vi "Observer.vi"(8 "Tau":dbl[](array[numeric]), 9 "y":dbl[](array[numeric]), 11 "OBS_K":dbl[](array[numeric])) -> (2 "q_hat":T1)   [LabVIEW 2019]
uses:
  <vilib>/Analysis/Matrix/Datatypes/RealMatrix.ctl
  <vilib>/Analysis/Matrix/NI_Matrix.lvlib
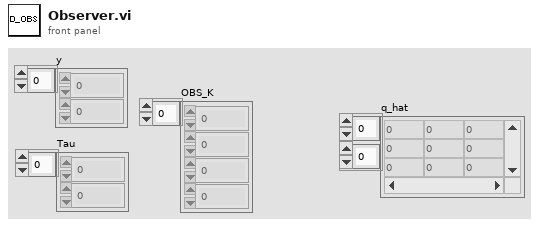
[diagram p1: front panel]
types:
  T1 = typedef "NI_Matrix.lvlib/RealMatrix.ctl" = dbl[][]
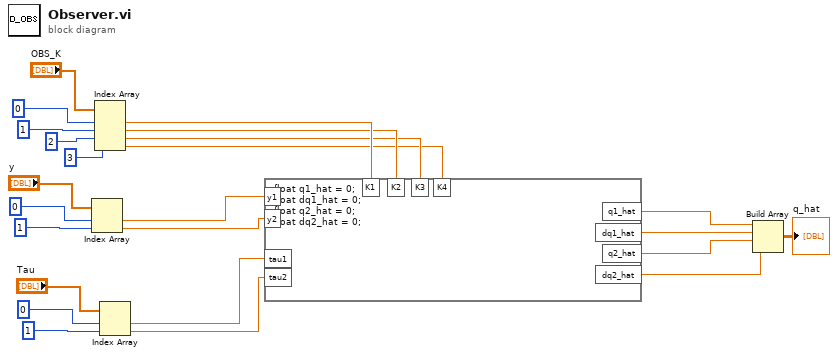
[diagram p0: block diagram]
diagram:
  n1 = Index Array(array="y", index #1=0 ("index (row)"), index #2=1 ("index (col)")) -> (element #1=w2:dbl, element #2=w1:dbl)
  n2 = Index Array(array="OBS_K", index #1=0 ("index (row)"), index #2=1 ("index (col)"), index #3=2 ("index"), index #4=3 ("index")) -> (element #1=w19:dbl, element #2=w18:dbl, element #3=w17:dbl, element #4=w16:dbl)
  n3 = Index Array(array="Tau", index #1=0 ("index (row)"), index #2=1 ("index (col)")) -> (element #1=w7:dbl, element #2=w6:dbl)
  n4 = formula code="float q1_hat = 0;\nfloat dq1_hat = 0;\nfloat q2_hat = 0;\nfloat dq2_hat = 0;"("y1"=w2, "K2"=w18, "K1"=w19, "K3"=w17, "K4"=w16, "tau1"=w7, "tau2"=w6, "y2"=w1) -> ("q1_hat"=w15:dbl, "dq1_hat"=w14:dbl, "q2_hat"=w13:dbl, "dq2_hat"=w12:dbl)
  n5 = Build Array(w15, w14, w13, w12) -> (→"q_hat":T1)
